vi "Measure Power Sample.vi"() -> ()   [LabVIEW 2023]
panel:
  out "Active":bool
  out "Power Value":dbl caption="Optical Power [W]" format="%#_4p"
  in  "stop":bool
  # "Thorlabs Power Meter Series\n   Measure power example"
  # "This example will connect the first found power meter."
  # "Connected"
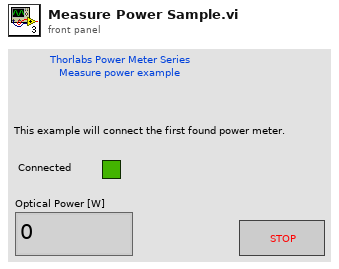
[diagram p1: front panel]
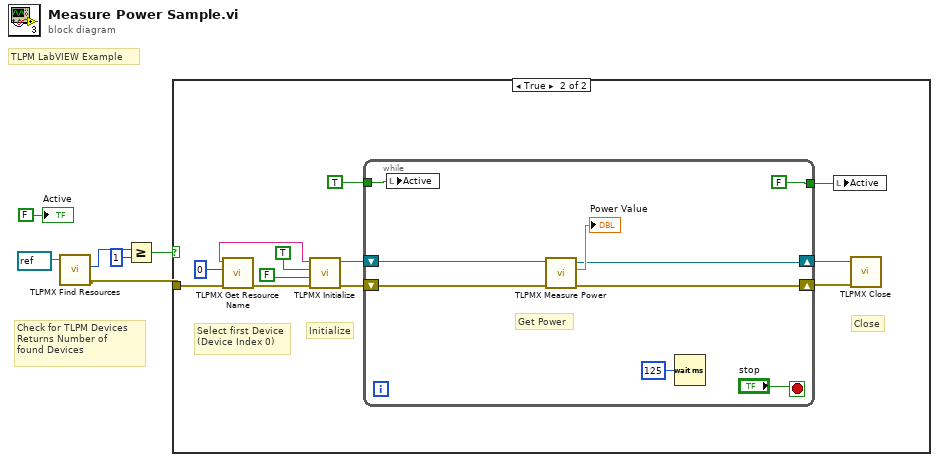
[diagram p0: block diagram]
diagram:
  # "TLPM LabVIEW Example"
  # "Check for TLPM Devices\nReturns Number of\nfound Devices"
  n1 = call <instrlib>:"TLPMX Find Resources.vi"("instrument handle"=refnum<visa-resource-name> refnum) -> ("error out"=w2:errorcluster, "Resource Count"=w1:u32)  [unwired: 8 in, 1 out]
  n2 = Greater Or Equal?(x=w1, y=u32 1) -> (x >= y?=w6:bool)
  n3 = case shown="True" w6 {
    tunnel: w2 -> [_ w13]
    frame False {
    }
    frame True {
      # "Close"
      # "Initialize"
      # "Select first Device\n(Device Index 0)"
      n4 = call <instrlib>:"TLPMX Get Resource Name.vi"("error in (no error)"=w13, "Index (0)"=u32 0 ("Device Index")) -> ("error out"=w9:errorcluster, "Resource Name"=w11:string)  [unwired: 7 in, 1 out]
      n5 = call <instrlib>:"TLPMX Initialize.vi"("error in (no error)"=w9, "Reset Device (Yes)"=FALSE ("ID Query (Do Query)"), "ID Query (Yes)"=TRUE ("ID Query (Do Query)"), "resource name"=w11) -> ("error out"=w7:errorcluster, "instrument handle out"=w8:refnum<visa-resource-name>)  [unwired: 6 in]
      n6 = while {
        shift-right: [w21] -> w16
        shift-left: w8 -> [w19]
        shift-right: [w22] -> w15
        shift-left: w7 -> [w20]
        tunnel: [FALSE ("Active")] -> w18
        tunnel: TRUE ("Active") -> [w24]
        stop <- "stop" stop-if-true
        # "Get Power"
        n7 = local write "Active"(w24) -> ()
        n8 = call <instrlib>:"TLPMX Measure Power.vi"("error in (no error)"=w20, "instrument handle"=w19) -> ("error out"=w22:errorcluster, "Power"=→"Power Value":dbl, "instrument handle out"=w21:refnum<visa-resource-name>)  [unwired: 7 in]
        n9 = Wait (ms)(milliseconds to wait=u32 125) -> ()  [unwired: 1 out]
      }
      n10 = local write "Active"(w18) -> ()
      n11 = call <instrlib>:"TLPMX Close.vi"("error in (no error)"=w15, "instrument handle"=w16) -> ()  [unwired: 9 in, 1 out]
    }
  }
  "Active" <- FALSE ("Active")
